vi "CAN_GetReceiveNum.vi"(8 "错误输入（无错误）":errorcluster, 11 "General_Input":T2) -> (0 "错误输出":errorcluster, 2 "GetReceiveNum":u32, 3 "General_Output":T1)   [LabVIEW 2012]
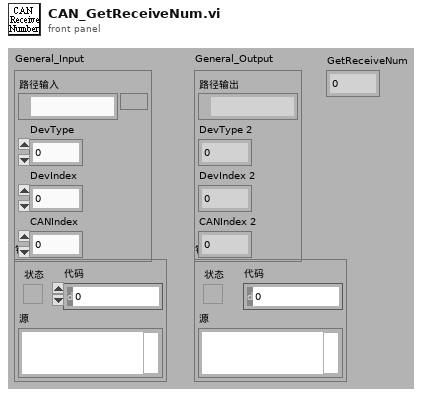
[diagram p1: front panel]
types:
  T1 = cluster{"路径输出":path, "DevType 2":u32, "DevIndex 2":u32, "CANIndex 2":u32}
  T2 = cluster{"路径输入":path, "DevType":u32, "DevIndex":u32, "CANIndex":u32}
  T3 = cluster{"path out":path, "DevType":u32, "DevIndex":u32, "CANIndex":u32}
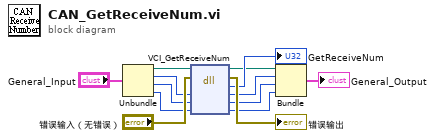
[diagram p0: block diagram]
diagram:
  n1 = Unbundle("General_Input") -> ("路径输入"=w9:path, "DevType"=w6:u32, "DevIndex"=w7:u32, "CANIndex"=w8:u32)
  n2 = dll-call lib="E:/1_Projects/ITMS/API Library/ControlCAN.dll" fn="VCI_GetReceiveNum"(path in=w9, error in="错误输入（无错误）", "DevType"=w6, "DevIndex"=w7, "CANIndex"=w8) -> (path out=w5:path, error out=→"错误输出":errorcluster, "GetReceiveNum"=→"GetReceiveNum":u32, "DevType"=w2:u32, "DevIndex"=w3:u32, "CANIndex"=w4:u32)  [unwired: 1 in]
  n3 = Bundle("path out"=w5, "DevType"=w2, "DevIndex"=w3, "CANIndex"=w4) -> (→"General_Output":T3)  [unwired: 1 in]
